vi "UI test.vi"() -> ()   [LabVIEW 2018]
uses:
  <vilib>/userdefined/High Color/IMAQdx.ctl
  <vilib>/vision/Image Controls.llb/IMAQ Image.ctl
  <vilib>/vision/driver/IMAQdx.llb/IMAQdx Acquisition Mode.ctl
  <vilib>/DAQmx/read.llb/DAQmx Read (Analog 1D Wfm NChan NSamp).vi
  support/Message Queue/Enqueue Message (Single).vi
  <vilib>/DAQmx/miscellaneous.llb/DAQmx Fill In Error Info.vi
  support/Message Queue/Message Queue.lvlib
  <vilib>/vision/driver/NI_Vision_Acquisition_Software.lvlib
  <resource>/objmgr/daqmx.rc
panel:
  out "就绪状态":bool=TRUE
  in  "Vertical Print Button":bool
  in  "Vertical Save Button":bool
  in  "Vertical Open Button":bool
  in  "Vertical HW Info Button":bool
  in  "Vertical Info Button":bool
  in  "Vertical Settings Button":bool
  in  "中间选项卡":enum32{"  设置  ", "  示波  ", "  分析  "}(tab)
  out "Image 4":T1(plugin-control)
  out "阵列形状：":cluster{dbl[], dbl[]}(graph)
  out "Image 6":T1(plugin-control)
  in  "选项卡控件 2":enum32{"设置", "示波", "分析"}(tab)
  in  "频段":enum16{""}(ring)
  in  "滤波":enum16{""}(ring)
  in  "算法":enum16{""}(ring)
  out "String (transparent)":string
  in  "阵型":enum16{""}(ring)
  in  "相机":enum16{""}(ring)
  in  "聚焦面":enum16{""}(ring)
  in  "选择阵列":enum16{"圆形阵列 32阵元"}(ring)
  in  "System Start Button":bool
  in  "System Stop Button":bool
  in  "分析":enum16{""}(ring)
  in  "分析2":enum16{""}(ring)
  in  "分析3":enum16{""}(ring)
  out "State":string
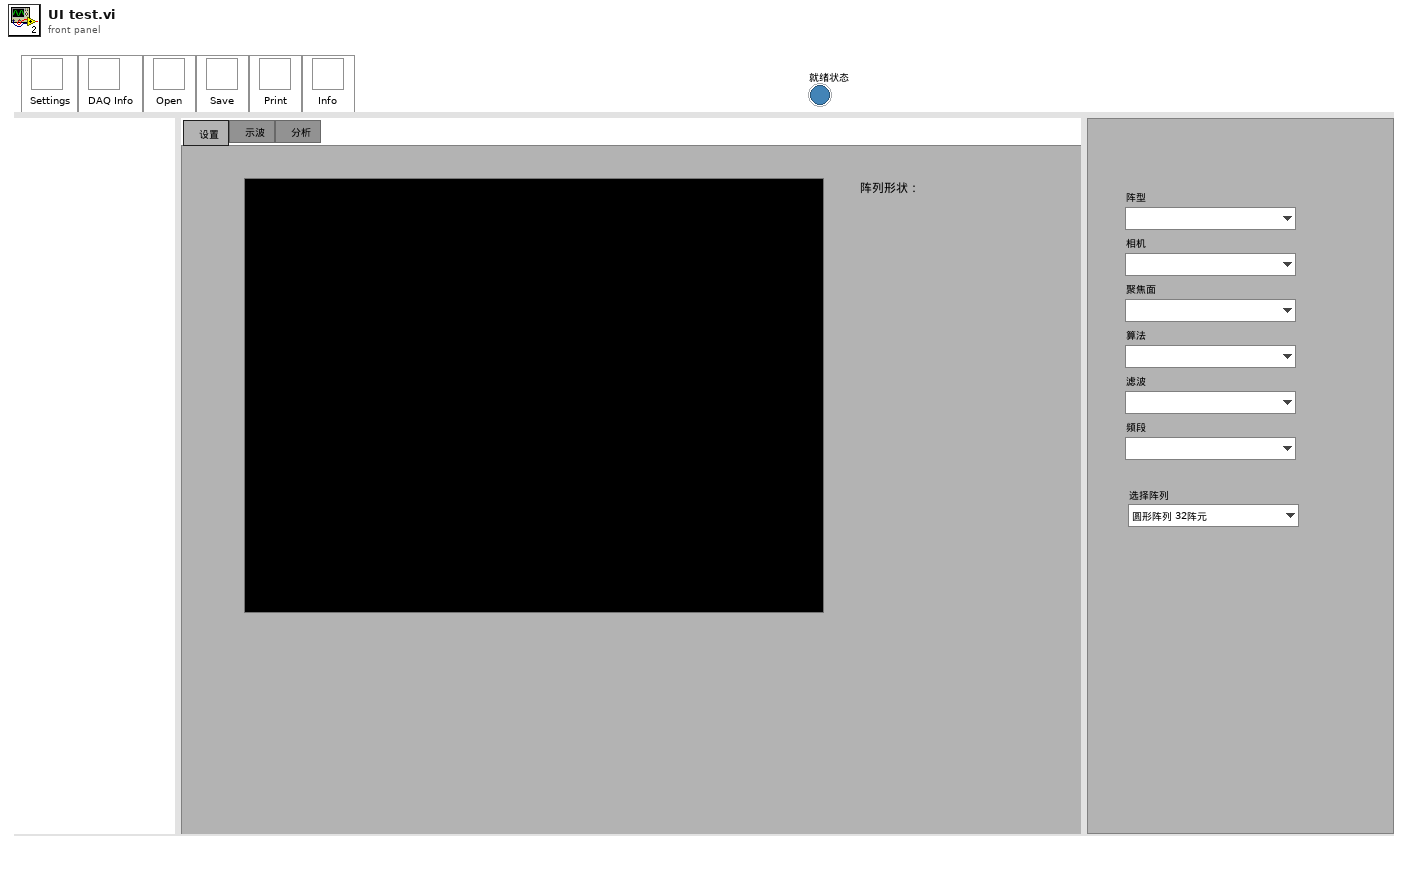
[diagram p1: front panel]
types:
  T1 = typedef "IMAQ Image.ctl" = refnum<image>
  T2 = typedef "IMAQdx.ctl" = refnum<k21>
  T3 = cluster{"Session In":T2, "State":enum16{"Stopped", "Running"}, "New Image":T1}
  T4 = cluster{"State":enum16{"Stopped", "Running"}, "DAQ AI Task":refnum<k21>}
  T5 = typedef "Message Queue.lvlib/All Message Queues.ctl" = cluster{"Marshaling Command":refnum<queue>, "UI Updata":refnum<queue>, "Processing Command":refnum<queue>, "DAQ Control":refnum<queue>, "Camera Control":refnum<queue>}
  T6 = typedef "NI_Vision_Acquisition_Software.lvlib/IMAQdx Acquisition Mode.ctl" = enum32{"One Shot", "Continuous"}
  T7 = typedef "Image Type" = u32
  T8 = cluster{"Type":u32, "Version":u32, "Flags":u32, "SerialNumberHigh":u32, "SerialNumberLow":u32, "BusType":u32, "InterfaceName":string, "VendorName":string, "ModelName":string, "CameraFileName":string, "CameraAttributeURL":string}[]
  T9 = cluster{"Type":u32, "Version":u32, "Flags":u32, "SerialNumberHigh":u32, "SerialNumberLow":u32, "BusType":u32, "InterfaceName":string, "VendorName":string, "ModelName":string, "CameraFileName":string, "CameraAttributeURL":string}
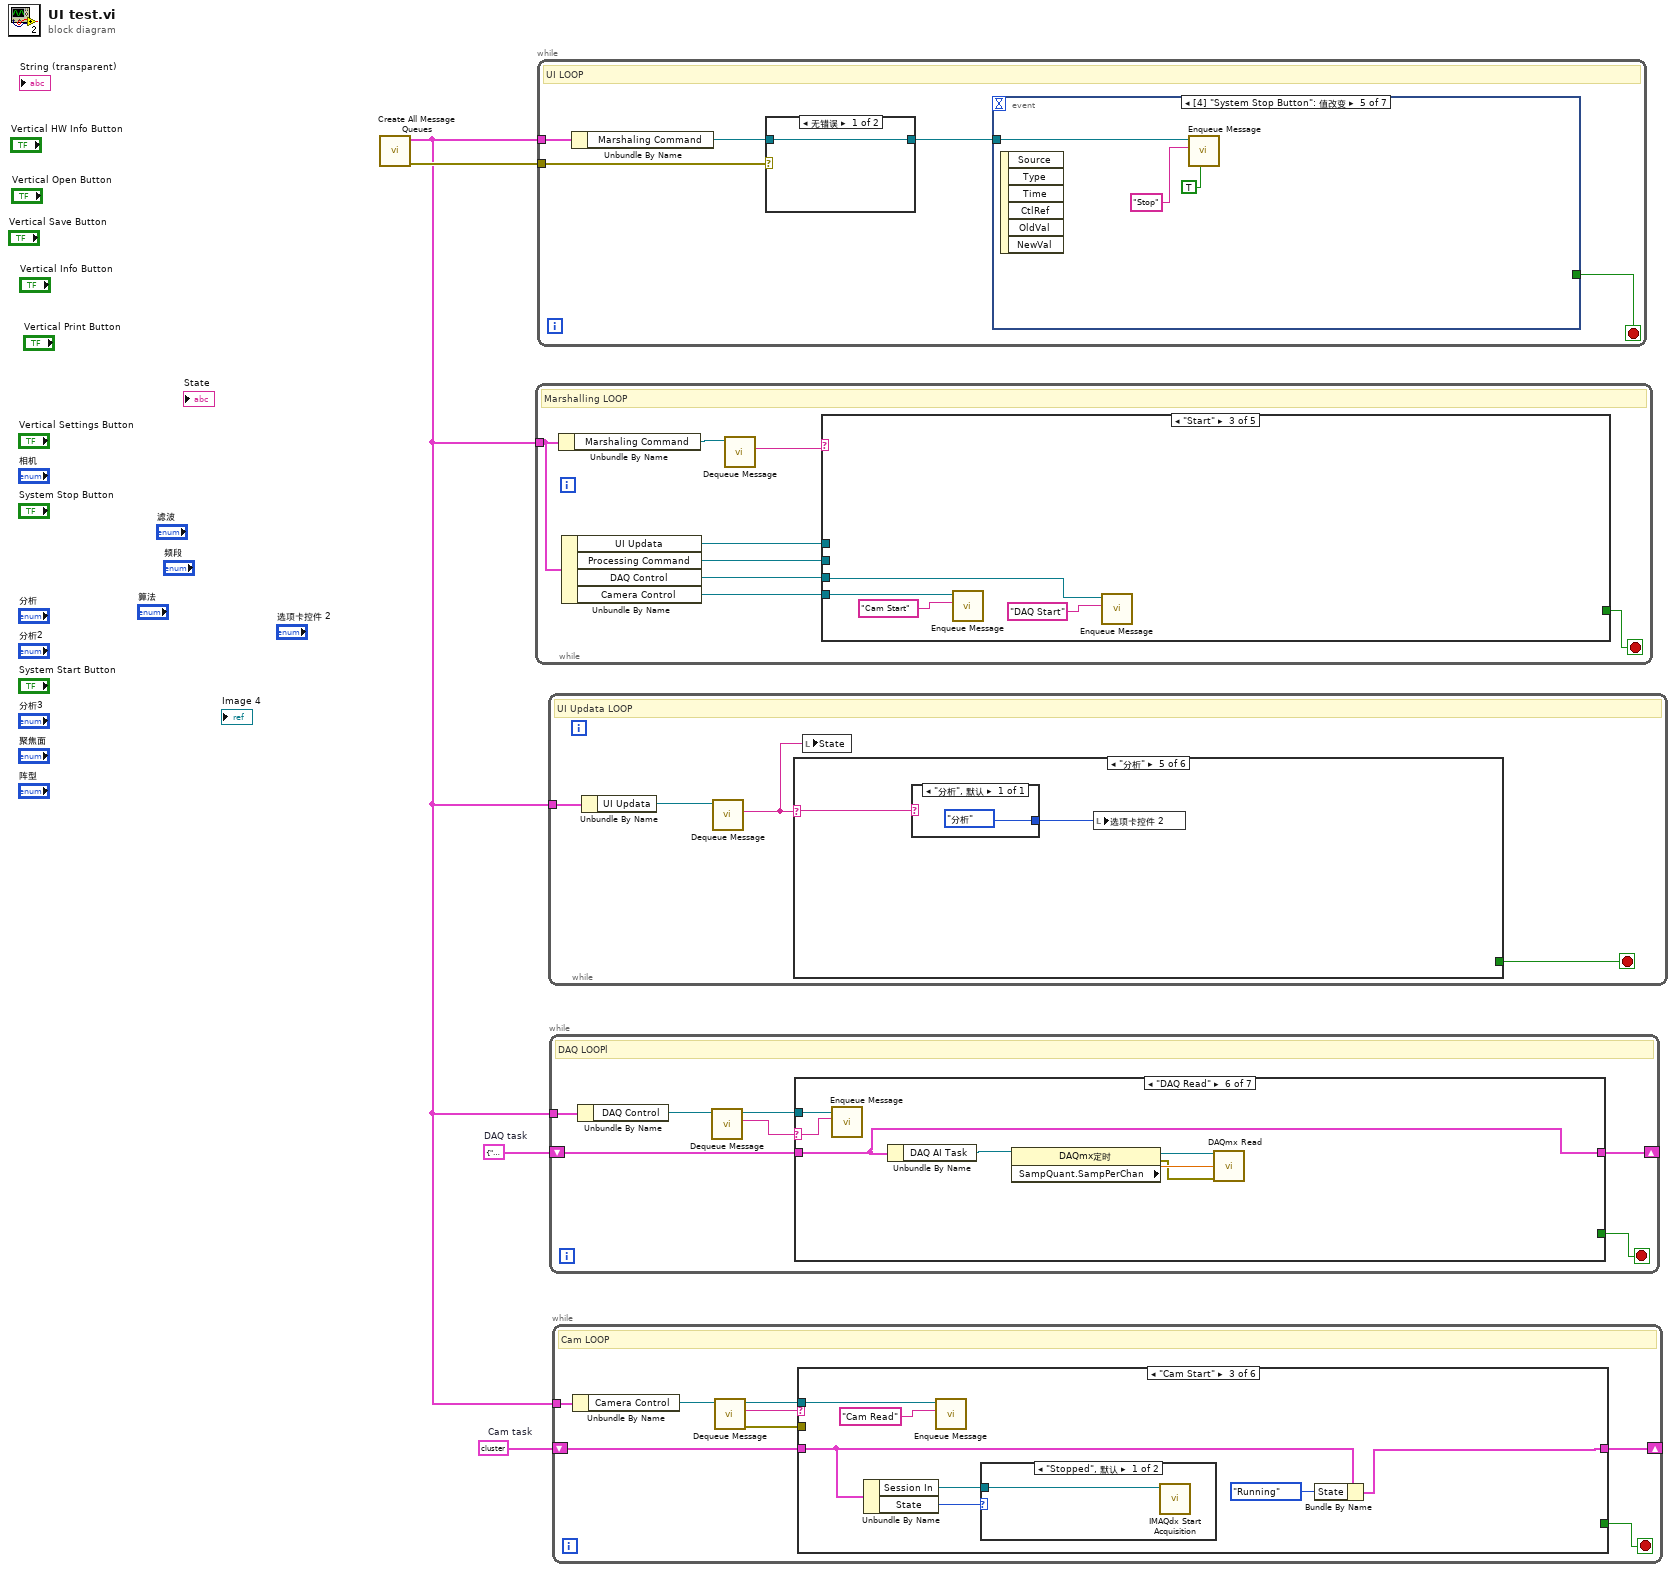
[diagram p0: block diagram]
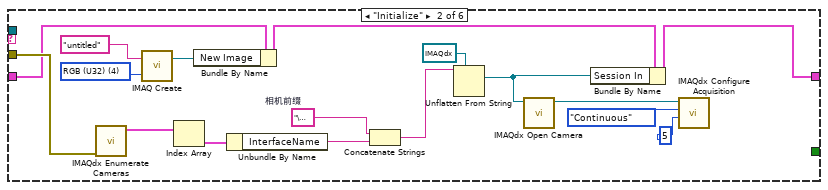
[diagram p3: hidden frame]
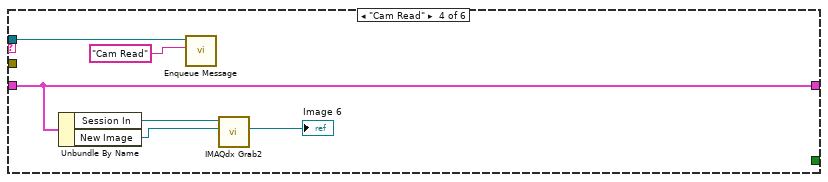
[diagram p5: hidden frame]
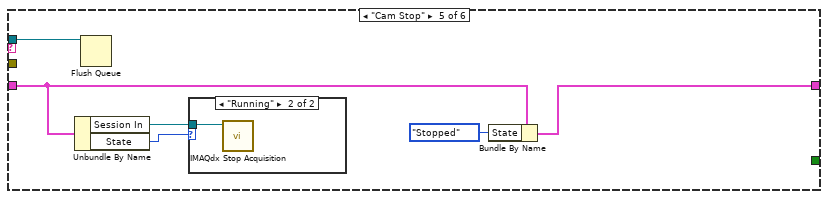
[diagram p6: hidden frame]
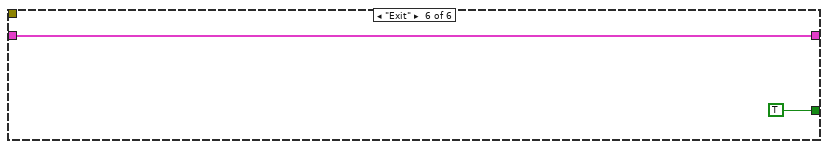
[diagram p8: hidden frame]
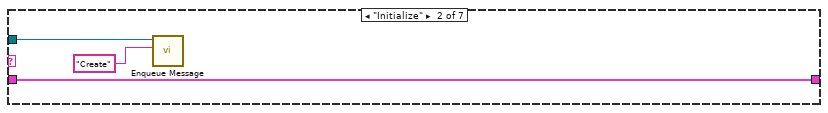
[diagram p10: hidden frame]
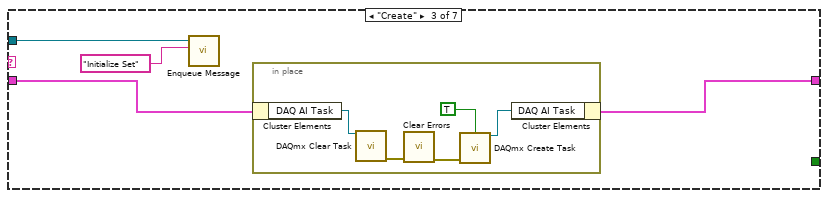
[diagram p11: hidden frame]
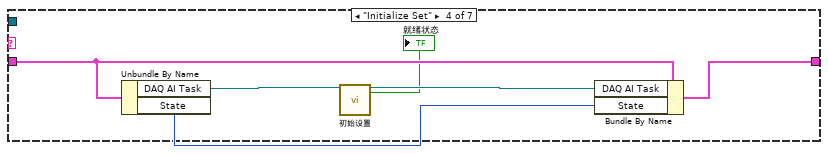
[diagram p12: hidden frame]
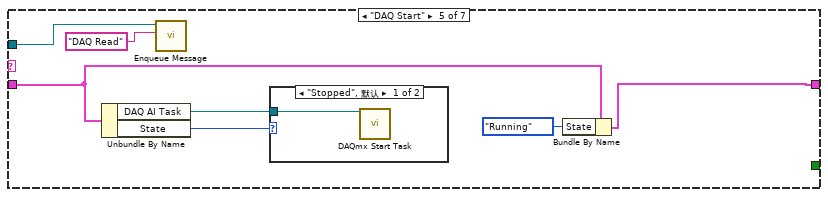
[diagram p13: hidden frame]
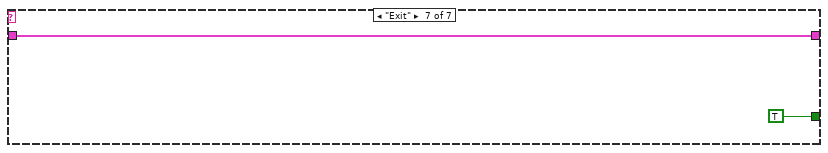
[diagram p15: hidden frame]
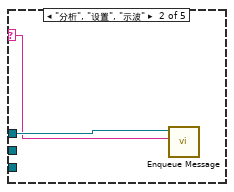
[diagram p17: hidden frame]
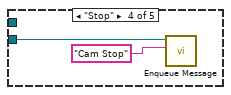
[diagram p18: hidden frame]
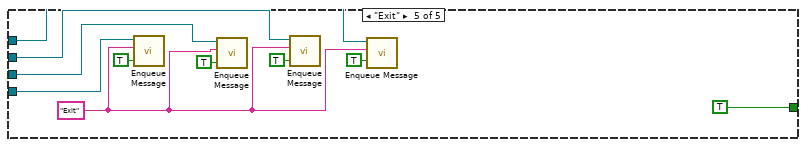
[diagram p19: hidden frame]
diagram:
  w1 = T3 {"Session In"="cam1", "State"=enum."Stopped", "New Image"=refnum}  # Cam task
  w2 = T4 {"State"=enum."Stopped", "DAQ AI Task"=""}  # DAQ task
  n1 = call "Create All Message Queues.vi"() -> ("error out"=w4:cluster{"状态":bool, "代码":i32, "源":string}, "消息队列输出"=w3:T5)  [unwired: 10 in]
  n2 = while {
    tunnel: w3 -> [w10]
    stop <- w9 stop-if-true
    # "Marshalling LOOP"
    n3 = Unbundle By Name(w10) -> ("Marshaling Command"=w12:refnum<queue>)
    n4 = Unbundle By Name(w10) -> ("UI Updata"=w8:refnum<queue>, "Processing Command"=w6:refnum<queue>, "DAQ Control"=w5:refnum<queue>, "Camera Control"=w7:refnum<queue>)
    n5 = call "Dequeue Message.vi"("消息队列"=w12) -> ("消息"=w11:string)  [unwired: 7 in, 3 out]
    n6 = case shown="\"Start\"" w11 {
      selector: w11 -> [_ w13 _ _ _]
      tunnel: [_ _ _ _ TRUE] -> w9
      tunnel: w8 -> [_ w14 _ _ w22]
      tunnel: w7 -> [_ _ w17 w19 w25]
      tunnel: w6 -> [_ _ _ _ w23]
      tunnel: w5 -> [_ _ w15 _ w24]
      frame "Wait", Default {
      }
      frame "分析", "设置", "示波" {
        n7 = call-poly "Enqueue Message.vi"("消息"=w13, "消息队列"=w14) -> ()  [unwired: 8 in, 2 out]
      }
      frame "Start" {
        n8 = call-poly "Enqueue Message.vi"("消息"="Cam Start", "消息队列"=w17) -> ()  [unwired: 8 in, 2 out]
        n9 = call-poly "Enqueue Message.vi"("消息"="DAQ Start", "消息队列"=w15) -> ()  [unwired: 8 in, 2 out]
      }
      frame "Stop" {
        n10 = call-poly "Enqueue Message.vi"("消息"="Cam Stop", "消息队列"=w19) -> ()  [unwired: 8 in, 2 out]
      }
      frame "Exit" {
        w21 = "Exit" ("消息")
        n11 = call-poly "Enqueue Message.vi"("优先消息？ (F)"=TRUE, "消息"=w21, "消息队列"=w25) -> ()  [unwired: 7 in, 2 out]
        n12 = call-poly "Enqueue Message.vi"("优先消息？ (F)"=TRUE, "消息"=w21, "消息队列"=w24) -> ()  [unwired: 7 in, 2 out]
        n13 = call-poly "Enqueue Message.vi"("优先消息？ (F)"=TRUE, "消息"=w21, "消息队列"=w23) -> ()  [unwired: 7 in, 2 out]
        n14 = call-poly "Enqueue Message.vi"("优先消息？ (F)"=TRUE, "消息"=w21, "消息队列"=w22) -> ()  [unwired: 7 in, 2 out]
      }
    }
  }
  n15 = while {
    tunnel: w3 -> [w34]
    tunnel: w4 -> [w33]
    stop <- w35 stop-if-true
    # "UI LOOP"
    n16 = Unbundle By Name(w34) -> ("Marshaling Command"=w32:refnum<queue>)
    n17 = case shown="无错误" w33 {
      selector: w33 -> [_ w38]
      tunnel: w32 -> [w36 w40]
      tunnel: [w36 w37] -> w31
      frame No Error {
      }
      frame Error {
        n18 = call-poly "Enqueue Message.vi"("error in (no error)"=w38, "消息"="Error Handle", "消息队列"=w40) -> ("消息队列副本"=w37:refnum<queue>)  [unwired: 7 in, 1 out]
      }
    }
    n19 = event shown="[4] \"System Stop Button\": 值改变" {
      selector: _ -> [_ _ _ _ _ _ _]
      dyn-events: _ -> [_ _ _ _ _ _ _]
      timeout: _ -> [_ _ _ _ _ _ _]
      tunnel: [_ _ _ _ _ TRUE TRUE] -> w35
      tunnel: w31 -> [_ _ w42 w48 w50 _ w55]
      event Timeout {
        n20 = event-data() -> ()  [unwired: 1 in, 3 out]
      }
      event "State": Value Change {
        n21 = event-data() -> ()  [unwired: 1 in, 4 out]
      }
      event "中间选项卡": Value Change {
        n22 = event-data() -> ("NewVal"=w43:enum32{"  设置  ", "  示波  ", "  分析  "})  [unwired: 1 in, 5 out]
        n23 = case shown="\"  分析  \"" w43 {
          tunnel: ["设置" "示波" "分析"] -> w41
          frame "  设置  ", Default {
          }
          frame "  示波  " {
          }
          frame "  分析  " {
          }
        }
        n24 = call-poly "Enqueue Message.vi"("消息"=w41, "消息队列"=w42) -> ()  [unwired: 8 in, 2 out]
      }
      event "System Start Button": Value Change {
        n25 = event-data() -> ()  [unwired: 1 in, 6 out]
        n26 = call-poly "Enqueue Message.vi"("消息"="Start", "消息队列"=w48) -> ()  [unwired: 8 in, 2 out]
      }
      event "System Stop Button": Value Change {
        n27 = event-data() -> ()  [unwired: 1 in, 6 out]
        n28 = call-poly "Enqueue Message.vi"("优先消息？ (F)"=TRUE, "消息"="Stop", "消息队列"=w50) -> ()  [unwired: 7 in, 2 out]
      }
      event Panel Close {
        n29 = event-data() -> ()  [unwired: 1 in, 4 out]
      }
      event "Vertical Save Button": Value Change {
        n30 = event-data() -> ()  [unwired: 1 in, 6 out]
        n31 = call-poly "Enqueue Message.vi"("优先消息？ (F)"=TRUE, "消息"="Exit", "消息队列"=w55) -> ()  [unwired: 7 in, 2 out]
      }
    }
  }
  n32 = while {
    tunnel: w3 -> [w59]
    stop <- w60 stop-if-true
    # "UI Updata LOOP"
    n33 = Unbundle By Name(w59) -> ("UI Updata"=w58:refnum<queue>)
    n34 = call "Dequeue Message.vi"("消息队列"=w58) -> ("消息"=w57:string)  [unwired: 7 in, 3 out]
    n35 = case shown="\"分析\"" w57 {
      selector: w57 -> [_ _ w66 w70 w73 _]
      tunnel: [_ _ _ _ _ TRUE] -> w60
      frame "假", Default {
      }
      frame "Initialize" {
        w65 = cluster{"颜色盒":u32, "颜色盒":u32} {"颜色盒"=16777238, "颜色盒"=16777238} ("簇")
        n36 = property on="分隔栏 3" class="Splitter"("Colors"=w65) -> ()  [unwired: 2 in, 2 out]
        n37 = property on="分隔栏 2" class="Splitter"("Colors"=w65) -> ()  [unwired: 2 in, 2 out]
        n38 = property on="分隔栏" class="Splitter"("Colors"=w65) -> ()  [unwired: 2 in, 2 out]
        n39 = property on="分隔栏 4" class="Splitter"("Colors"=w65) -> ()  [unwired: 2 in, 2 out]
        n40 = local write "选项卡控件 2"(enum32{"设置", "示波", "分析"}."设置" ("选项卡控件 2")) -> ()
        n41 = local write "中间选项卡"(enum32{"  设置  ", "  示波  ", "  分析  "}."  设置  " ("中间选项卡")) -> ()
        n42 = call "阵型选择.vi"("选择阵列"="选择阵列") -> ("阵列形状："=→"阵列形状：":cluster{dbl[], dbl[]})  [unwired: 18 in]
      }
      frame "设置" {
        n43 = case shown="\"设置\", 默认" w66 {
          tunnel: [enum32{"设置", "示波", "分析"}."设置" ("选项卡控件 2")] -> w67
          frame "设置", Default {
          }
        }
        n44 = local write "选项卡控件 2"(w67) -> ()
      }
      frame "示波" {
        n45 = case shown="\"示波\", 默认" w70 {
          tunnel: [enum32{"设置", "示波", "分析"}."示波" ("选项卡控件 2")] -> w69
          frame "示波", Default {
          }
        }
        n46 = local write "选项卡控件 2"(w69) -> ()
      }
      frame "分析" {
        n47 = case shown="\"分析\", 默认" w73 {
          tunnel: [enum32{"设置", "示波", "分析"}."分析" ("选项卡控件 2")] -> w72
          frame "分析", Default {
          }
        }
        n48 = local write "选项卡控件 2"(w72) -> ()
      }
      frame "Exit" {
      }
    }
    n49 = local write "State"(w57) -> ()
  }
  n50 = while {
    tunnel: w3 -> [w82]
    shift-right: [w77] -> _
    shift-left: w2 -> [w78]
    stop <- w79 stop-if-true
    # "DAQ LOOPl"
    n51 = Unbundle By Name(w82) -> ("DAQ Control"=w81:refnum<queue>)
    n52 = call "Dequeue Message.vi"("消息队列"=w81) -> ("消息"=w80:string, "消息队列副本"=w76:refnum<queue>)  [unwired: 7 in, 2 out]
    n53 = case shown="\"DAQ Read\"" w80 {
      selector: w80 -> [_ _ _ _ _ w110 _]
      tunnel: [_ _ _ _ _ _ TRUE] -> w79
      tunnel: w78 -> [w83 w84 w90 w100 w106 w114 w117]
      tunnel: [w83 w84 w89 w98 w105 w114 w117] -> w77
      tunnel: w76 -> [_ w86 w87 _ w103 w111 _]
      frame "Wait", Default {
      }
      frame "Initialize" {
        n54 = call-poly "Enqueue Message.vi"("消息"="Create", "消息队列"=w86) -> ()  [unwired: 8 in, 2 out]
      }
      frame "Create" {
        n55 = call-poly "Enqueue Message.vi"("消息"="Initialize Set", "消息队列"=w87) -> ()  [unwired: 8 in, 2 out]
        n56 = in-place {
          n57 = in-place-cluster #1(w90) -> ("DAQ AI Task"=w95:refnum<k21>)
          n58 = call <vilib>:"DAQmx Clear Task.vi"("task in"=w95) -> ("error out"=w94:errorcluster)  [unwired: 14 in]
          n59 = call <vilib>:"Clear Errors.vi"("error in (no error)"=w94) -> ("error out"=w93:errorcluster)  [unwired: 5 in, 1 out]
          n60 = call <vilib>:"DAQmx Create Task.vi"("auto cleanup"=TRUE, "error in"=w93) -> ("task out"=w92:refnum<k21>)  [unwired: 12 in, 1 out]
          n61 = in-place-cluster #1("DAQ AI Task"=w92) -> (w89:T4)
        }
      }
      frame "Initialize Set" {
        n62 = Unbundle By Name(w100) -> ("DAQ AI Task"=w101:refnum<k21>, "State"=w97:enum16{"Stopped", "Running"})
        n63 = call "初始设置.vi"("引用句柄输入"=w101) -> ("就绪状态"=→"就绪状态":bool, "task out"=w99:refnum<k21>)  [unwired: 16 in, 1 out]
        n64 = Bundle By Name(cluster=w100, "DAQ AI Task"=w99, "State"=w97) -> (w98:T4)
      }
      frame "DAQ Start" {
        n65 = Unbundle By Name(w106) -> ("DAQ AI Task"=w107:refnum<k21>, "State"=w108:enum16{"Stopped", "Running"})
        n66 = call-poly "Enqueue Message.vi"("消息"="DAQ Read", "消息队列"=w103) -> ()  [unwired: 8 in, 2 out]
        n67 = case shown="\"Stopped\", 默认" w108 {
          tunnel: w107 -> [w109 _]
          frame "Stopped", Default {
            n68 = call <vilib>:"DAQmx Start Task.vi"("task/channels in"=w109) -> ()  [unwired: 13 in, 2 out]
          }
          frame "Running" {
          }
        }
        n69 = Bundle By Name(cluster=w106, "State"=enum16{"Stopped", "Running"}."Running") -> (w105:T4)
      }
      frame "DAQ Read" {
        n70 = call-poly "Enqueue Message.vi"("消息"=w110, "消息队列"=w111) -> ()  [unwired: 8 in, 2 out]
        n71 = Unbundle By Name(w114) -> ("DAQ AI Task"=w113:refnum<k21>)
        n72 = property class="DAQmx定时"(reference=w113) -> (reference out=w112:refnum<k21>, error out=w115:errorcluster, "SampQuant.SampPerChan"=w116:dbl)  [unwired: 1 in]
        n73 = call-poly <vilib>:"DAQmx Read.vi"("task/channels in"=w112, "number of samples per channel"=w116, "error in"=w115) -> ()  [unwired: 10 in, 3 out]
      }
      frame "Exit" {
      }
    }
  }
  n74 = while {
    tunnel: w3 -> [w126]
    shift-right: [w121] -> _
    shift-left: w1 -> [w122]
    stop <- w123 stop-if-true
    # "Cam LOOP"
    n75 = Unbundle By Name(w126) -> ("Camera Control"=w125:refnum<queue>)
    n76 = call "Dequeue Message.vi"("消息队列"=w125) -> ("error out"=w120:cluster{"状态":bool, "代码":i32, "源":string}, "消息"=w124:string, "消息队列副本"=w119:refnum<queue>)  [unwired: 7 in, 1 out]
    n77 = case shown="\"Cam Start\"" w124 {
      tunnel: [_ _ _ _ _ TRUE] -> w123
      tunnel: w122 -> [w127 w134 w147 w156 w161 w166]
      tunnel: [w127 w131 w145 w156 w160 w166] -> w121
      tunnel: w120 -> [_ w144 _ _ _ _]
      tunnel: w119 -> [_ _ w149 w153 w162 _]
      frame "Wait", Default {
      }
      frame "Initialize" {
        w135 = T7 4 items=["Grayscale (U8)", "Grayscale (I16)", "Grayscale (SGL)", "Complex (CSG)", "RGB (U32)", "HSL (U32)", "RGB (U64)", "Grayscale (U16)"] ("Image Type")
        w141 = "\u0000\u0000\u0000\u0004"  # 相机前缀
        n78 = call <vilib>:"IMAQdx Enumerate Cameras.vi"("error in"=w144) -> ("Camera Information Array"=w143:T8)  [unwired: 9 in, 1 out]
        n79 = call "IMAQ Create"("Image Name"="untitled", "Image Type"=w135) -> ("New Image"=w133:T1)  [unwired: 3 in, 1 out]
        n80 = Index Array(array=w143) -> (element=w142:T9)  [unwired: 1 in]
        n81 = Bundle By Name(cluster=w134, "New Image"=w133) -> (w132:T3)
        n82 = Unbundle By Name(w142) -> ("InterfaceName"=w140:string)
        n83 = Concatenate Strings(w141, w140) -> (w139:string)
        n84 = Unflatten From String(type=T2 refnum ("Session In"), binary string=w139) -> (value=w137:T2)  [unwired: 3 in, 2 out]
        n85 = call <vilib>:"IMAQdx Open Camera.vi"("Session In"=w137) -> ("Session Out"=w129:T2)  [unwired: 9 in, 1 out]
        n86 = Bundle By Name(cluster=w132, "Session In"=w137) -> (w131:T3)
        n87 = call <vilib>:"IMAQdx Configure Acquisition.vi"("Number of Buffers"=u32 5, "Continuous?"=IMAQdx_Acquisition_Mode."Continuous", "Session In"=w129) -> ()  [unwired: 7 in, 2 out]
      }
      frame "Cam Start" {
        n88 = Unbundle By Name(w147) -> ("Session In"=w151:T2, "State"=w148:enum16{"Stopped", "Running"})
        n89 = call-poly "Enqueue Message.vi"("消息"="Cam Read", "消息队列"=w149) -> ()  [unwired: 8 in, 2 out]
        n90 = case shown="\"Stopped\", 默认" w148 {
          tunnel: w151 -> [w152 _]
          frame "Stopped", Default {
            n91 = call <vilib>:"IMAQdx Start Acquisition.vi"("Session In"=w152) -> ()  [unwired: 9 in, 2 out]
          }
          frame "Running" {
          }
        }
        n92 = Bundle By Name(cluster=w147, "State"=enum16{"Stopped", "Running"}."Running") -> (w145:T3)
      }
      frame "Cam Read" {
        n93 = Unbundle By Name(w156) -> ("Session In"=w158:T2, "New Image"=w155:T1)
        n94 = call-poly "Enqueue Message.vi"("消息"="Cam Read", "消息队列"=w153) -> ()  [unwired: 8 in, 2 out]
        n95 = call <vilib>:"IMAQdx Grab2.vi"("Image In"=w155, "Session In"=w158) -> ("Image Out"=→"Image 6":T1)  [unwired: 6 in, 3 out]
      }
      frame "Cam Stop" {
        n96 = Unbundle By Name(w161) -> ("Session In"=w164:T2, "State"=w163:enum16{"Stopped", "Running"})
        n97 = Flush Queue(queue=w162) -> ()  [unwired: 1 in, 3 out]
        n98 = case shown="\"Running\"" w163 {
          tunnel: w164 -> [_ w165]
          frame "Stopped", Default {
          }
          frame "Running" {
            n99 = call <vilib>:"IMAQdx Stop Acquisition.vi"("Session In"=w165) -> ()  [unwired: 9 in, 2 out]
          }
        }
        n100 = Bundle By Name(cluster=w161, "State"=enum16{"Stopped", "Running"}."Stopped") -> (w160:T3)
      }
      frame "Exit" {
      }
    }
  }
